vi "LAb4gui.vi"() -> ()   [LabVIEW 2026]
uses:
  led_toggle/Serial - Settings.ctl
  <vilib>/Instr/_visa.llb/VISA Flush IO Buffer Mask.ctl
  <vilib>/Instr/_visa.llb/VISA Configure Serial Port (Instr).vi
panel:
  out "Indicators":T1
  in  "Controls":T2 {"Detection Threshold" scale=0.0..500.0; "Blur" scale=0.0..100.0}
  out "error out":errorcluster
  in  "COM Port":refnum<visa-resource-name>
  in  "Serial Settings":T3={"baud rate"=115200, "data bits"=8, "parity"=enum."None", "stop bits"=10, "flow control"=0} {"flow control" items=["None"=0, "XON/XOFF"=1, "RTS/CTS"=2, "DTR/DSR"=4]; "stop bits" items=["1.0"=10, "1.5"=15, "2.0"=20]; "data bits" min=5 max=8 step=1; "baud rate" items=["75"=75, "110"=110, "134"=134, "150"=150, "300"=300, "600"=600, "1200"=1200, "1800"=1800, "2400"=2400, "4800"=4800, "7200"=7200, "9600"=9600, "14400"=14400, "19200"=19200, "28800"=28800, "38400"=38400, "56000"=56000, "57600"=57600, "115200"=115200, "128000"=128000, "230400"=230400]}
  in  "stop":bool
  in  "Send Filters":bool
  in  "Reset Filters":bool
  in  "Display ON/OFF":bool
  in  "Get Status":bool
  # "DISPLAY"
  # "DEVICE STATUS"
  # "IMAGE FILTERS"
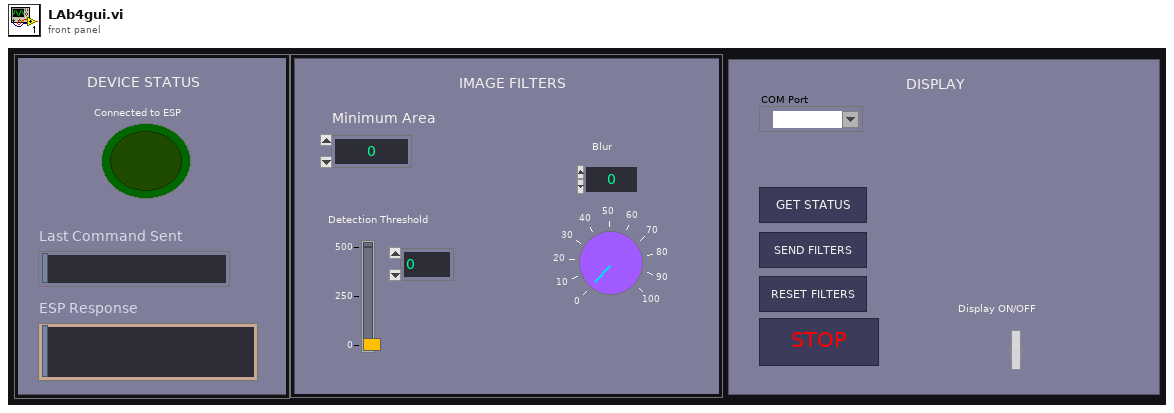
[diagram p1: front panel]
types:
  T1 = cluster{"Connected to ESP":bool, "Last Command Sent":string, "ESP Response":string}
  T2 = cluster{"Minimum Area  ":i32, "Blur":i32, "Detection Threshold ":i32}
  T3 = typedef "Serial - Settings.ctl" = cluster{"baud rate":u32, "data bits":u16, "parity":enum16{"None", "Odd", "Even", "Mark", "Space"}, "stop bits":u16, "flow control":u16}
  T4 = cluster{"Controls":cluster{"Minimum Area  ":i32, "Blur":i32, "Detection Threshold ":i32}, "Indicators":cluster{"Connected to ESP":bool, "Last Command Sent":string, "ESP Response":string}}
  T5 = enum16{"Init", "Connect", "Idle", "Get Status", "Display ON", "Display OFF", "Send Filters", "Reset Filters", "Read Reply", "Error", "Stop"}
  T6 = typedef "VISA Flush IO Buffer Mask.ctl" = u16
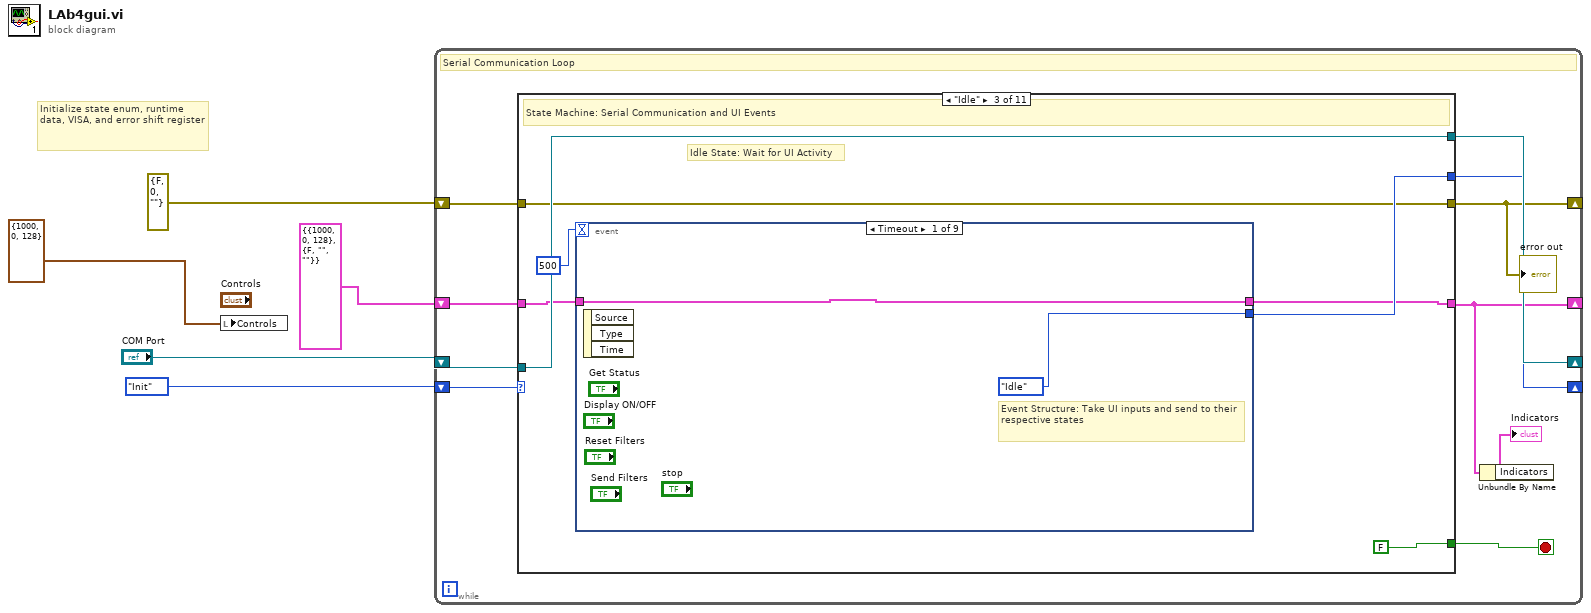
[diagram p0: block diagram]
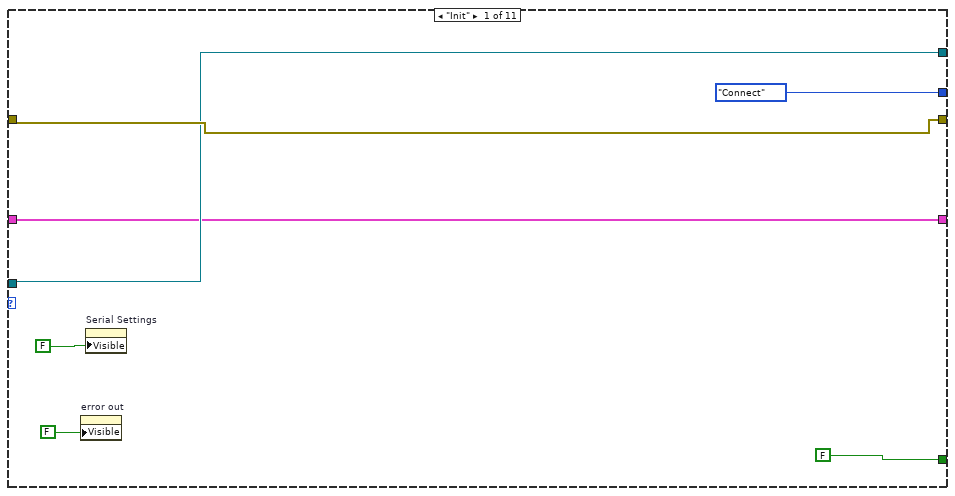
[diagram p2: hidden frame]
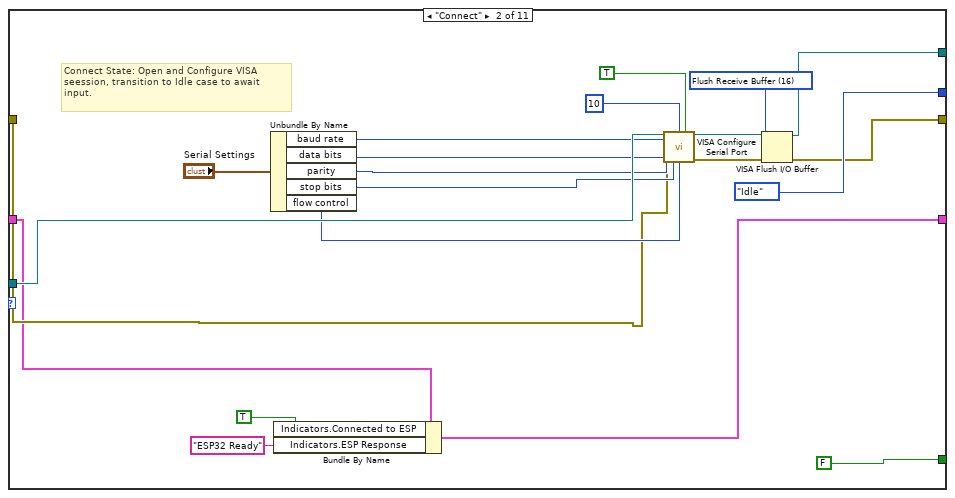
[diagram p3: hidden frame]
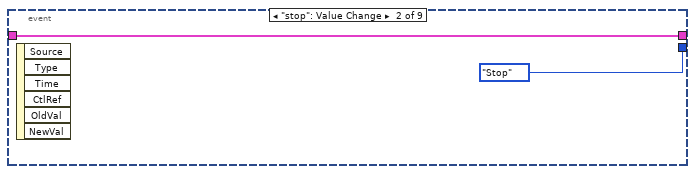
[diagram p4: hidden frame]
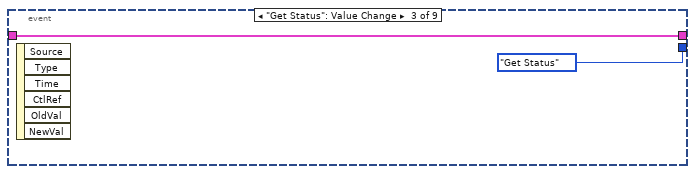
[diagram p5: hidden frame]
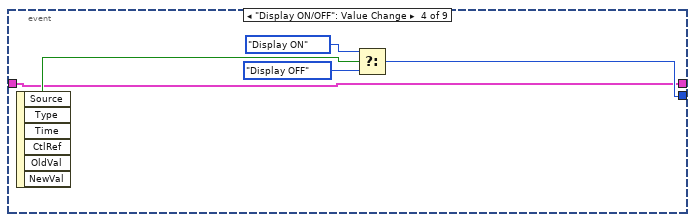
[diagram p6: hidden frame]
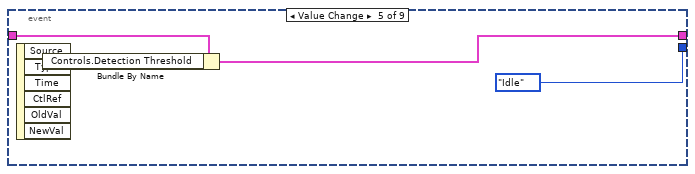
[diagram p7: hidden frame]
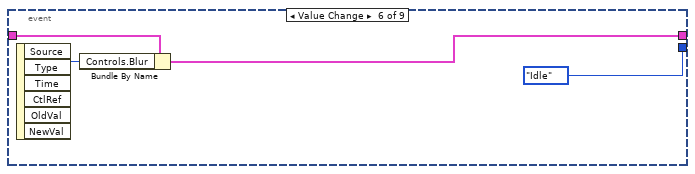
[diagram p8: hidden frame]
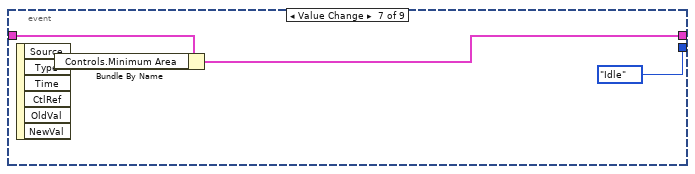
[diagram p9: hidden frame]
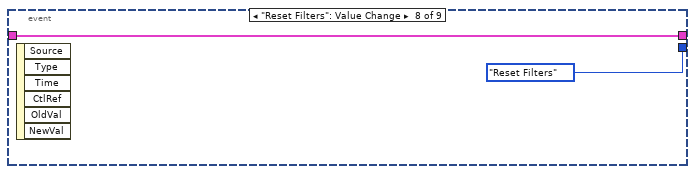
[diagram p10: hidden frame]
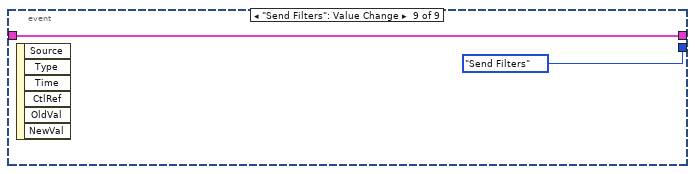
[diagram p11: hidden frame]
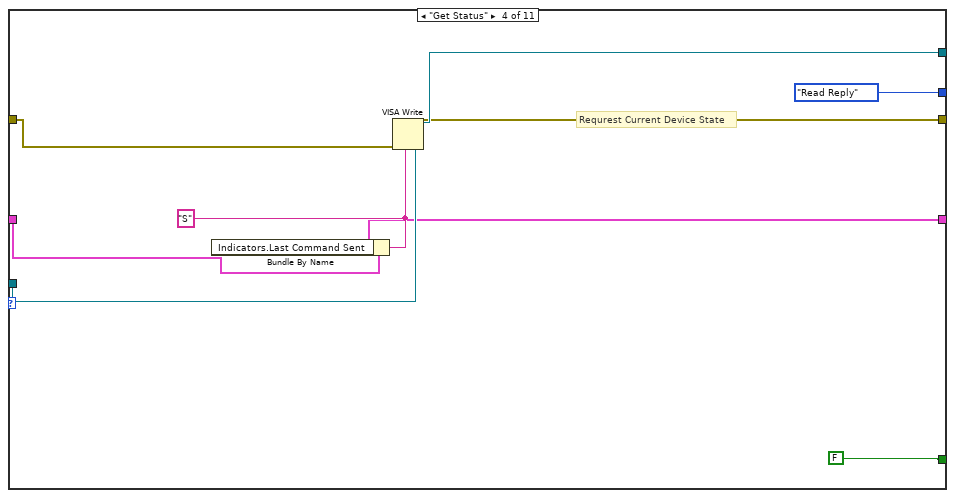
[diagram p12: hidden frame]
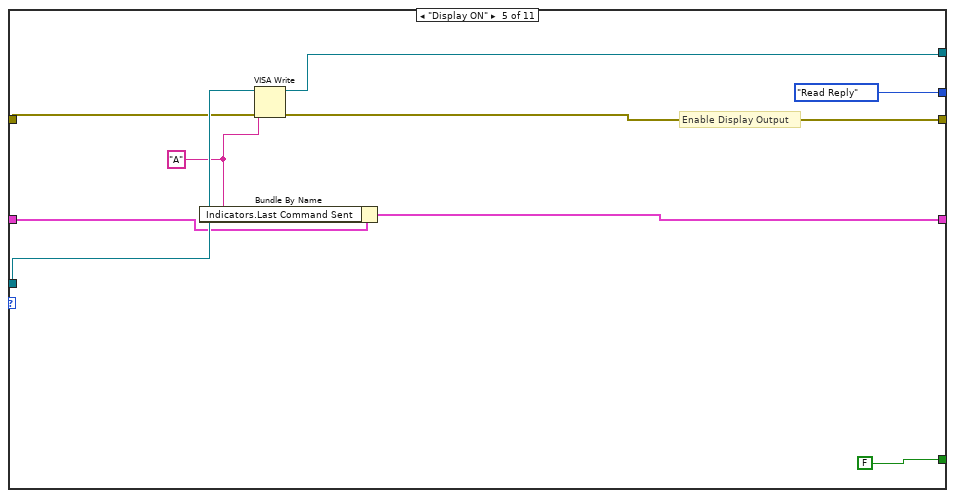
[diagram p13: hidden frame]
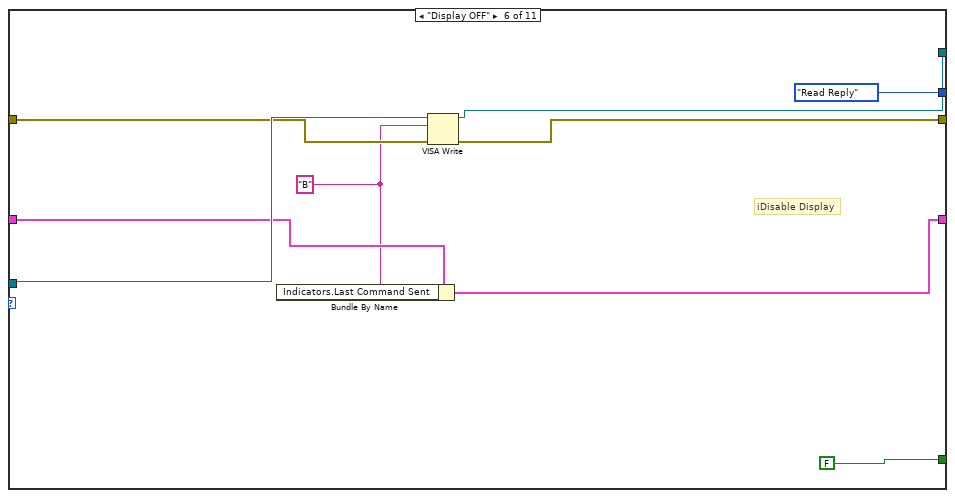
[diagram p14: hidden frame]
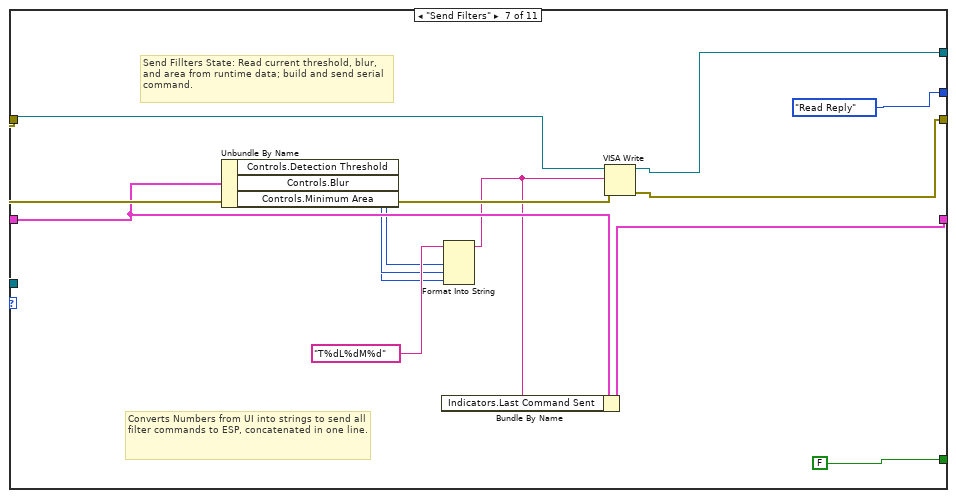
[diagram p15: hidden frame]
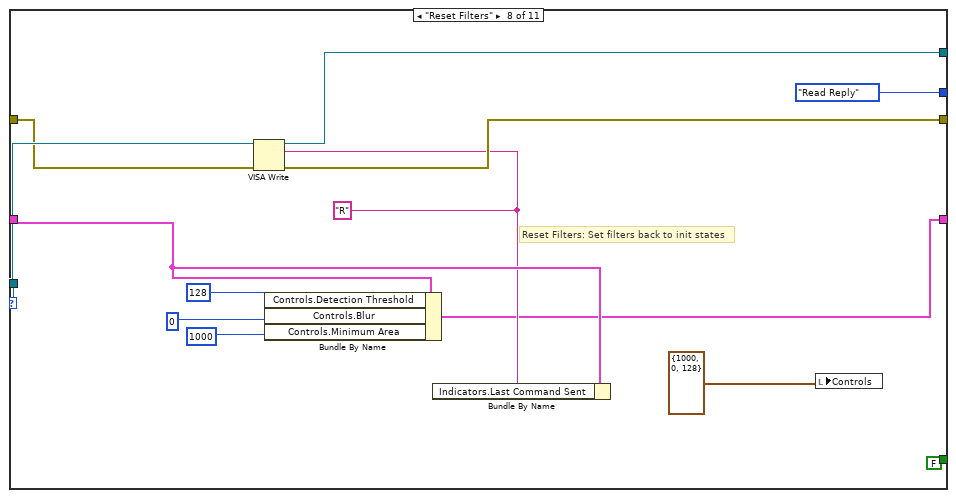
[diagram p16: hidden frame]
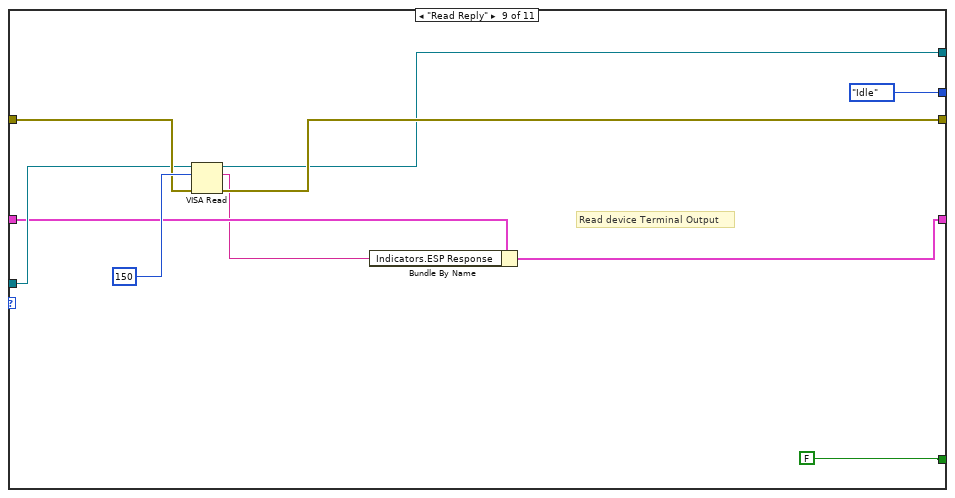
[diagram p17: hidden frame]
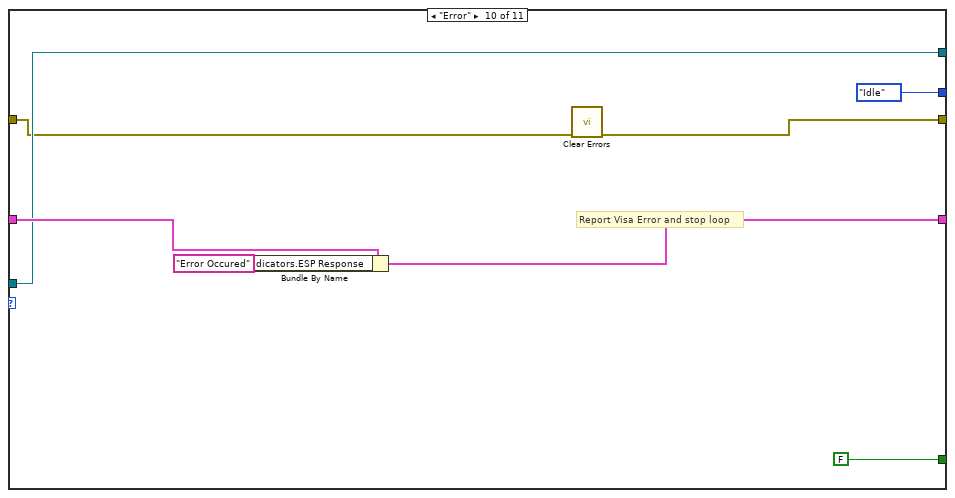
[diagram p18: hidden frame]
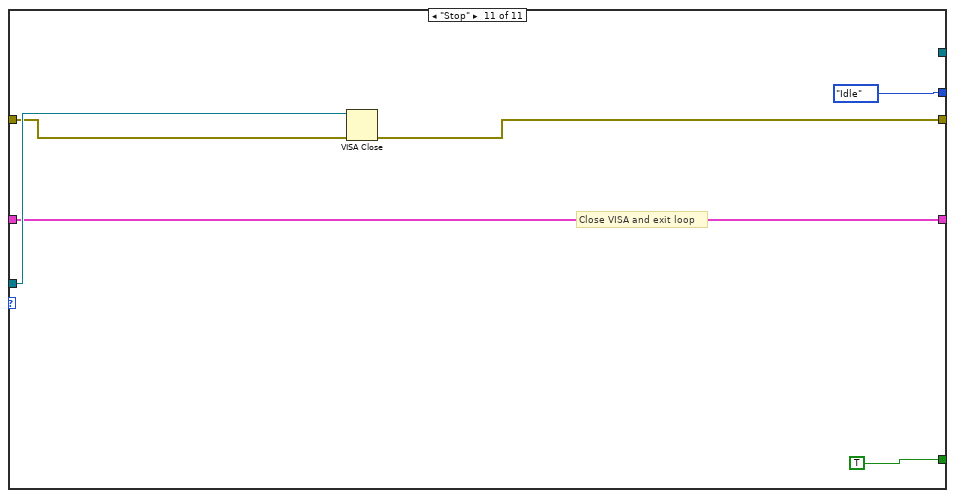
[diagram p19: hidden frame]
diagram:
  # "Initialize state enum, runtime data, VISA, and error shift register"
  n1 = local write "Controls"(T2 {"Minimum Area  "=1000, "Blur"=0, "Detection Threshold "=128} ("Controls")) -> ()
  n2 = while {
    shift-right: [w13] -> _
    shift-left: T5."Init" -> [w15]
    shift-right: [w14] -> _
    shift-left: "COM Port" -> [w6]
    shift-right: [w10] -> _
    shift-left: errorcluster {"status"=FALSE, "code"=0, "source"=""} ("error out") -> [w12]
    shift-right: [w7] -> _
    shift-left: T4 {"Controls"={"Minimum Area  "=1000, "Blur"=0, "Detection Threshold "=128}, "Indicators"={"Connected to ESP"=FALSE, "Last Command Sent"="", "ESP Response"=""}} -> [w9]
    stop <- w11 stop-if-true
    # "Serial Communication Loop"
    n3 = case shown="\"Idle\"" w15 {
      tunnel: [w21 w28 w49 w84 w92 w101 w106 w128 w137 w143 _] -> w14
      tunnel: [w22 w27 w47 w82 w91 w102 w105 w127 w138 w141 w151] -> w10
      tunnel: [T5."Connect" T5."Idle" w48 T5."Read Reply" T5."Read Reply" T5."Read Reply" T5."Read Reply" T5."Read Reply" T5."Idle" T5."Idle" T5."Idle"] -> w13
      tunnel: w12 -> [w22 w35 w47 w85 w94 w103 w116 w129 w135 w142 w152]
      tunnel: w6 -> [w21 w41 w49 w86 w95 w104 w117 w130 w134 w143 w153]
      tunnel: [FALSE FALSE FALSE FALSE FALSE FALSE FALSE FALSE FALSE FALSE TRUE] -> w11
      tunnel: w9 -> [w18 w32 w45 w80 w89 w98 w112 w122 w133 w146 w149]
      tunnel: [w18 w31 w44 w78 w87 w96 w113 w119 w131 w144 w149] -> w7
      frame "Init" {
        n4 = property on="error out" class="Clust (strict)"("Visible"=FALSE) -> ()  [unwired: 2 in, 2 out]
        n5 = property on="Serial Settings" class="Clust (strict)"("Visible"=FALSE) -> ()  [unwired: 2 in, 2 out]
      }
      frame "Connect" {
        w26 = T6 16 items=["Flush Receive Buffer"=16, "Write Transmit Buffer to Device"=32, "Flush Receive Buffer (No I/O)"=64, "Flush Transmit Buffer"=128] ("Mask")
        # "Connect State: Open and Configure VISA seession, transition to Idle case to await input."
        n6 = Unbundle By Name("Serial Settings") -> ("baud rate"=w40:u32, "data bits"=w39:u16, "parity"=w38:enum16{"None", "Odd", "Even", "Mark", "Space"}, "stop bits"=w37:u16, "flow control"=w36:u16)
        n7 = Bundle By Name(cluster=w32, "Indicators.Connected to ESP"=TRUE ("Connected to ESP"), "Indicators.ESP Response"="ESP32 Ready") -> (w31:T4)
        n8 = call-poly "VISA Configure Serial Port"("VISA resource name"=w41, "termination char\n(0xA = '\\n' = LF)"=u8 10 ("termination char\n(0xA = '\\n' = LF)"), "Enable Termination\nChar (T)"=TRUE ("Enable Termination\nChar (T)"), "baud rate (9600)"=w40, "data bits (8)"=w39, "parity (0:none)"=w38, "error in (no error)"=w35, "stop bits (10: 1 bit)"=w37, "flow control (0:none)"=w36) -> ("VISA resource name out"=w25:refnum<visa-resource-name>, "error out"=w24:errorcluster)  [unwired: 5 in]
        n9 = VISA Flush I/O Buffer(VISA resource name=w25, mask (16)=w26, error in (no error)=w24) -> (VISA resource name out=w28:refnum<visa-resource-name>, error out=w27:errorcluster)
      }
      frame "Idle" {
        # "Idle State: Wait for UI Activity"
        # "State Machine: Serial Communication and UI Events"
        n10 = event shown="[0] Timeout" {
          selector: _ -> [_ _ _ _ _ _ _ _ _]
          dyn-events: _ -> [_ _ _ _ _ _ _ _ _]
          timeout: 500 -> [_ _ _ _ _ _ _ _ _]
          tunnel: [T5."Idle" T5."Stop" T5."Get Status" w58 T5."Idle" T5."Idle" T5."Idle" T5."Reset Filters" T5."Send Filters"] -> w48
          tunnel: w45 -> [w51 w53 w55 w57 w64 w68 w72 w74 w76]
          tunnel: [w51 w53 w55 w57 w62 w66 w70 w74 w76] -> w44
          event Timeout {
            # "Event Structure: Take UI inputs and send to their respective states"
            n11 = event-data() -> ()  [unwired: 1 in, 3 out]
          }
          event "stop": Value Change {
            n12 = event-data() -> ()  [unwired: 1 in, 6 out]
          }
          event "Get Status": Value Change {
            n13 = event-data() -> ()  [unwired: 1 in, 6 out]
          }
          event "Display ON/OFF": Value Change {
            n14 = event-data() -> ("NewVal"=w61:bool)  [unwired: 1 in, 5 out]
            n15 = Select(t=T5."Display ON", s=w61, f=T5."Display OFF") -> (s? t:f=w58:T5)
          }
          event "Controls.Detection Threshold": Value Change {
            n16 = event-data() -> ("NewVal"=w63:i32)  [unwired: 1 in, 5 out]
            n17 = Bundle By Name(cluster=w64, "Controls.Detection Threshold"=w63) -> (w62:T4)
          }
          event "Controls.Blur": Value Change {
            n18 = event-data() -> ("NewVal"=w67:i32)  [unwired: 1 in, 5 out]
            n19 = Bundle By Name(cluster=w68, "Controls.Blur"=w67) -> (w66:T4)
          }
          event "Controls.Minimum Area": Value Change {
            n20 = event-data() -> ("NewVal"=w71:i32)  [unwired: 1 in, 5 out]
            n21 = Bundle By Name(cluster=w72, "Controls.Minimum Area"=w71) -> (w70:T4)
          }
          event "Reset Filters": Value Change {
            n22 = event-data() -> ()  [unwired: 1 in, 6 out]
          }
          event "Send Filters": Value Change {
            n23 = event-data() -> ()  [unwired: 1 in, 6 out]
          }
        }
      }
      frame "Get Status" {
        w79 = "S"
        # "Requrest Current Device State"
        n24 = Bundle By Name(cluster=w80, "Indicators.Last Command Sent"=w79) -> (w78:T4)
        n25 = VISA Write(VISA resource name=w86, write buffer=w79, error in (no error)=w85) -> (VISA resource name out=w84:refnum<visa-resource-name>, error out=w82:errorcluster)  [unwired: 1 out]
      }
      frame "Display ON" {
        w88 = "A"
        # "Enable Display Output"
        n26 = Bundle By Name(cluster=w89, "Indicators.Last Command Sent"=w88) -> (w87:T4)
        n27 = VISA Write(VISA resource name=w95, write buffer=w88, error in (no error)=w94) -> (VISA resource name out=w92:refnum<visa-resource-name>, error out=w91:errorcluster)  [unwired: 1 out]
      }
      frame "Display OFF" {
        w97 = "B"
        # "iDisable Display"
        n28 = Bundle By Name(cluster=w98, "Indicators.Last Command Sent"=w97) -> (w96:T4)
        n29 = VISA Write(VISA resource name=w104, write buffer=w97, error in (no error)=w103) -> (VISA resource name out=w101:refnum<visa-resource-name>, error out=w102:errorcluster)  [unwired: 1 out]
      }
      frame "Send Filters" {
        # "Converts Numbers from UI into strings to send all filter commands to ESP, concatenated in one line."
        # "Send Fillters State: Read current threshold, blur, and area from runtime data; build and send serial command."
        n30 = Unbundle By Name(w112) -> ("Controls.Detection Threshold"=w110:i32, "Controls.Blur"=w109:i32, "Controls.Minimum Area"=w108:i32)
        n31 = Format Into String(format string="T%dL%dM%d", w110, w109, w108) -> (resulting string=w107:string)  [unwired: 2 in, 1 out]
        n32 = Bundle By Name(cluster=w112, "Indicators.Last Command Sent"=w107) -> (w113:T4)
        n33 = VISA Write(VISA resource name=w117, write buffer=w107, error in (no error)=w116) -> (VISA resource name out=w106:refnum<visa-resource-name>, error out=w105:errorcluster)  [unwired: 1 out]
      }
      frame "Reset Filters" {
        w121 = "R" ("write buffer")
        # "Reset Filters: Set filters back to init states"
        n34 = VISA Write(VISA resource name=w130, write buffer=w121, error in (no error)=w129) -> (VISA resource name out=w128:refnum<visa-resource-name>, error out=w127:errorcluster)  [unwired: 1 out]
        n35 = Bundle By Name(cluster=w122, "Controls.Detection Threshold"=128 ("Detection Threshold"), "Controls.Blur"=0 ("Blur"), "Controls.Minimum Area"=1000 ("Minimum Area")) -> (w119:T4)
        n36 = Bundle By Name(cluster=w122, "Indicators.Last Command Sent"=w121) -> ()  [unwired: 1 out]
        n37 = local write "Controls"(T2 {"Minimum Area  "=1000, "Blur"=0, "Detection Threshold "=128} ("Controls")) -> ()
      }
      frame "Read Reply" {
        # "Read device Terminal Output"
        n38 = VISA Read(VISA resource name=w134, byte count=u32 150, error in (no error)=w135) -> (VISA resource name out=w137:refnum<visa-resource-name>, read buffer=w132:string, error out=w138:errorcluster)  [unwired: 1 out]
        n39 = Bundle By Name(cluster=w133, "Indicators.ESP Response"=w132) -> (w131:T4)
      }
      frame "Error" {
        # "Report Visa Error and stop loop"
        n40 = Bundle By Name(cluster=w146, "Indicators.ESP Response"="Error Occured") -> (w144:T4)
        n41 = call <vilib>:"Clear Errors.vi"("error in (no error)"=w142) -> ("error out"=w141:errorcluster)  [unwired: 5 in, 1 out]
      }
      frame "Stop" {
        # "Close VISA and exit loop"
        n42 = VISA Close(VISA resource name=w153, error in (no error)=w152) -> (error out=w151:errorcluster)
      }
    }
    "error out" <- w10
    n43 = Unbundle By Name(w7) -> ("Indicators"=→"Indicators":T1)
  }
